vi "GetSelected.vi"(8 "error in":errorcluster, 11 "Table Prefix":string="330AutonomousSelector") -> (0 "error out":errorcluster, 3 "Selected Autonomous Mode":string)   [LabVIEW 2012, in "AutonomousSelector.lvlib"]
doc: "Returns the selected Autonomous mode. If no Autonomous Mode is selected, the default is returned.\n\n<B>Table Prefix</B> The Sub Table in Network Tables. The data will be stored in /SmartDashboard/<Table Prefix>\n<B>Selected Autonomous Mode</B>The Selected Autonomous Mode"
uses:
  AutonomousSelector.lvlib
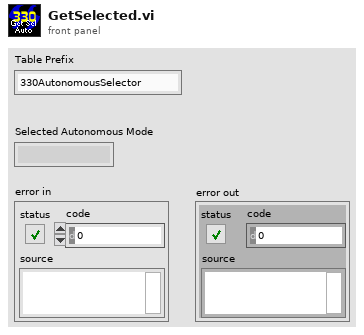
[diagram p1: front panel]
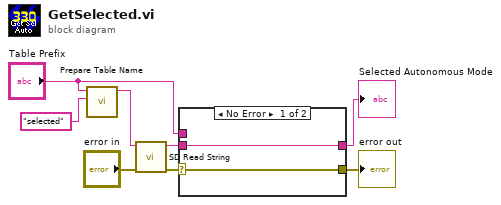
[diagram p0: block diagram]
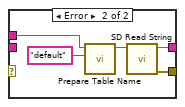
[diagram p2: hidden frame]
diagram:
  n1 = call <vilib>:"Prepare Table Name.vi"("Name"="selected", "Table Prefix"="Table Prefix") -> ("Prefixed Name"=w7:string)  [unwired: 9 in]
  n2 = call <vilib>:"SD Read String.vi"("error in"="error in", "Name"=w7) -> ("error out"=w6:errorcluster, "String"=w5:string)  [unwired: 7 in, 1 out]
  n3 = case shown="No Error" w6 {
    selector: w6 -> [w9 _]
    tunnel: [w10 w12] -> w4
    tunnel: w5 -> [w10 _]
    tunnel: "Table Prefix" -> [_ w14]
    tunnel: [w9 w11] -> w2
    frame No Error {
    }
    frame Error {
      n4 = call <vilib>:"Prepare Table Name.vi"("Name"="default", "Table Prefix"=w14) -> ("Prefixed Name"=w15:string)  [unwired: 9 in]
      n5 = call <vilib>:"SD Read String.vi"("Name"=w15) -> ("error out"=w11:errorcluster, "String"=w12:string)  [unwired: 8 in, 1 out]
    }
  }
  "Selected Autonomous Mode" <- w4
  "error out" <- w2
